vi "Esercitazione 3 - Esercizio per casa, enum giorno-mese.vi"() -> ()   [LabVIEW 2018]
panel:
  out "Non valido":bool
  in  "Mese":i32
  in  "Giorno":i32
  out "Valido":bool
  # "indicare se la coppia giorno-mese è una data valida nel calendario del 2020"
  # "suggerimento= enum, in range and coerce"
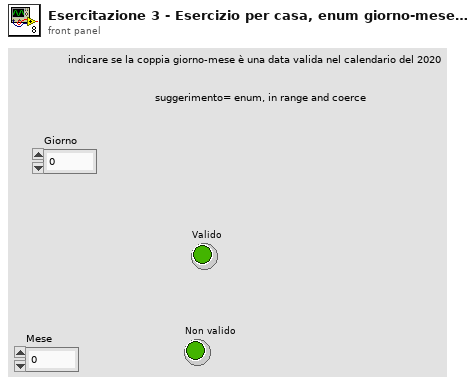
[diagram p1: front panel]
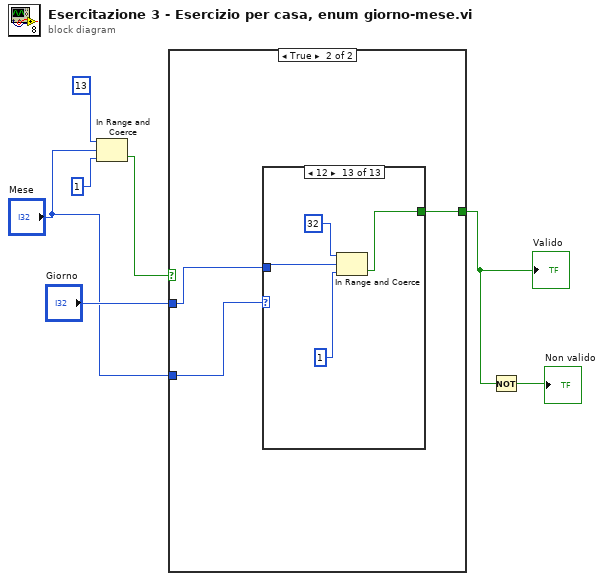
[diagram p0: block diagram]
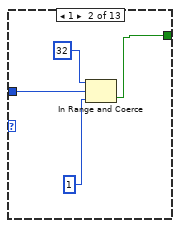
[diagram p4: hidden frame]
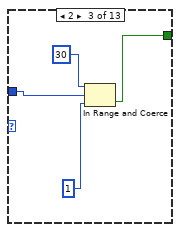
[diagram p5: hidden frame]
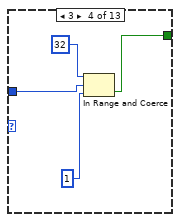
[diagram p6: hidden frame]
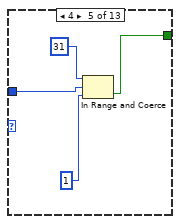
[diagram p7: hidden frame]
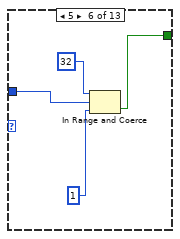
[diagram p8: hidden frame]
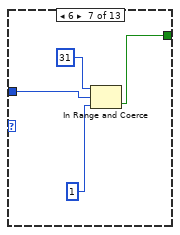
[diagram p9: hidden frame]
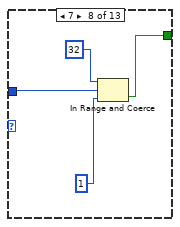
[diagram p10: hidden frame]
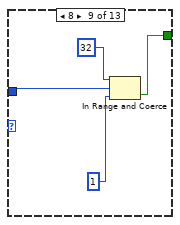
[diagram p11: hidden frame]
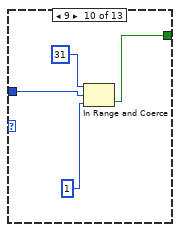
[diagram p12: hidden frame]
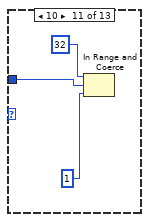
[diagram p13: hidden frame]
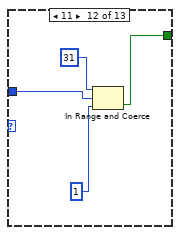
[diagram p14: hidden frame]
diagram:
  n1 = In Range and Coerce(upper limit=13, x="Mese", lower limit=1) -> (In Range?=w5:bool)  [unwired: 1 out]
  n2 = case shown="True" w5 {
    selector: w5 -> [w8 _]
    tunnel: [w8 w11] -> w1
    tunnel: "Giorno" -> [_ w9]
    tunnel: "Mese" -> [_ w10]
    frame False {
    }
    frame True {
      n3 = case shown="12" w10 {
        tunnel: [_ w13 w16 w20 w24 w28 w32 w36 w40 w44 _ w51 w55] -> w11
        tunnel: w9 -> [_ w12 w17 w21 w25 w29 w33 w37 w41 w45 w48 w52 w56]
        frame 0, Default {
        }
        frame 1 {
          n4 = In Range and Coerce(upper limit=32, x=w12, lower limit=1) -> (In Range?=w13:bool)  [unwired: 1 out]
        }
        frame 2 {
          n5 = In Range and Coerce(upper limit=30, x=w17, lower limit=1) -> (In Range?=w16:bool)  [unwired: 1 out]
        }
        frame 3 {
          n6 = In Range and Coerce(upper limit=32, x=w21, lower limit=1) -> (In Range?=w20:bool)  [unwired: 1 out]
        }
        frame 4 {
          n7 = In Range and Coerce(upper limit=31, x=w25, lower limit=1) -> (In Range?=w24:bool)  [unwired: 1 out]
        }
        frame 5 {
          n8 = In Range and Coerce(upper limit=32, x=w29, lower limit=1) -> (In Range?=w28:bool)  [unwired: 1 out]
        }
        frame 6 {
          n9 = In Range and Coerce(upper limit=31, x=w33, lower limit=1) -> (In Range?=w32:bool)  [unwired: 1 out]
        }
        frame 7 {
          n10 = In Range and Coerce(upper limit=32, x=w37, lower limit=1) -> (In Range?=w36:bool)  [unwired: 1 out]
        }
        frame 8 {
          n11 = In Range and Coerce(upper limit=32, x=w41, lower limit=1) -> (In Range?=w40:bool)  [unwired: 1 out]
        }
        frame 9 {
          n12 = In Range and Coerce(upper limit=31, x=w45, lower limit=1) -> (In Range?=w44:bool)  [unwired: 1 out]
        }
        frame 10 {
          n13 = In Range and Coerce(upper limit=32, x=w48, lower limit=1) -> ()  [unwired: 2 out]
        }
        frame 11 {
          n14 = In Range and Coerce(upper limit=31, x=w52, lower limit=1) -> (In Range?=w51:bool)  [unwired: 1 out]
        }
        frame 12 {
          n15 = In Range and Coerce(upper limit=32, x=w56, lower limit=1) -> (In Range?=w55:bool)  [unwired: 1 out]
        }
      }
    }
  }
  "Valido" <- w1
  n16 = Not(x=w1) -> (.not. x?=→"Non valido":bool)
